vi "Execute PID Controllers.vi"(8 "error in (no error)":errorcluster, 11 "State Variables in":T1 {"Config"."Config"."Industrial Settings"."Write Refs"."Data Reference" format="%.0x"; "Config"."Config"."Industrial Settings"."Read Refs"."Data Reference" format="%.0x"; "Config"."Config"."PID Settings"."Read Refs"."Data Reference" format="%.0x"; "Config"."Config"."PID Settings"."Write Refs"."Data Reference" format="%.0x"}) -> (0 "error out":errorcluster, 3 "State Variables out":T1 {"Config"."Config"."Industrial Settings"."Write Refs"."Data Reference" format="%.0x"; "Config"."Config"."Industrial Settings"."Read Refs"."Data Reference" format="%.0x"; "Config"."Config"."PID Settings"."Read Refs"."Data Reference" format="%.0x"; "Config"."Config"."PID Settings"."Write Refs"."Data Reference" format="%.0x"})   [LabVIEW 2019, in "Control Addon Engine.lvlib"]
uses:
  Control Addon Engine.lvlib
  Types/RT Driver State Variables.ctl
  <vilib>/NI/NIVS Inline Async API/_VS Inline Async API/VS Inline Async API/VS Inline Async API.lvclass
  Types/RT Configuration.ctl
  Addon Shared/Types/Gain Schedule.ctl
  Addon Shared/Types/Compiled Settings.ctl
  Addon Shared/Types/Compiled PID Settings.ctl
  <vilib>/NI VeriStand/Custom Device API/Block Data Reference.ctl
  <vilib>/NI VeriStand/Custom Device API/Data Reference.ctl
  Addon Shared/Types/Compiled Industrial Settings.ctl
  Addon Shared/Types/Compiled Industrial Parameters.ctl
  <vilib>/addons/control/pid/pid.llb/PID Parameter Manager (DBL Array).vi
  <vilib>/addons/control/pid/pid.llb/PID Derivative Action Buffered (DBL Array).vi
  <vilib>/addons/control/pid/pid.llb/PID Get Advanced Error (DBL Array).vi
  <vilib>/addons/control/pid/pid.llb/PID Integral Action Buffered (DBL Array).vi
  <vilib>/addons/control/pid/pid.llb/PID Resize 1D Array.vi
  <vilib>/addons/control/pid/pid.llb/PID Get Advanced Error (DBL).vi
  <vilib>/NI VeriStand/Custom Device API/Global Data Refs.vi
  <vilib>/addons/control/pid/pid.llb/PID Gain Schedule.vi
  <vilib>/addons/control/pid/pid.llb/PID Gain Schedule (DBL).vi
  <vilib>/addons/control/pid/pid.llb/PID Output Rate Limiter (DBL Array).vi
  <vilib>/NI VeriStand/Custom Device API/Custom Device API.lvlib
  <vilib>/addons/control/pid/NI_PID_pid.lvlib
  Addon Shared/Control Addon Shared.lvlib
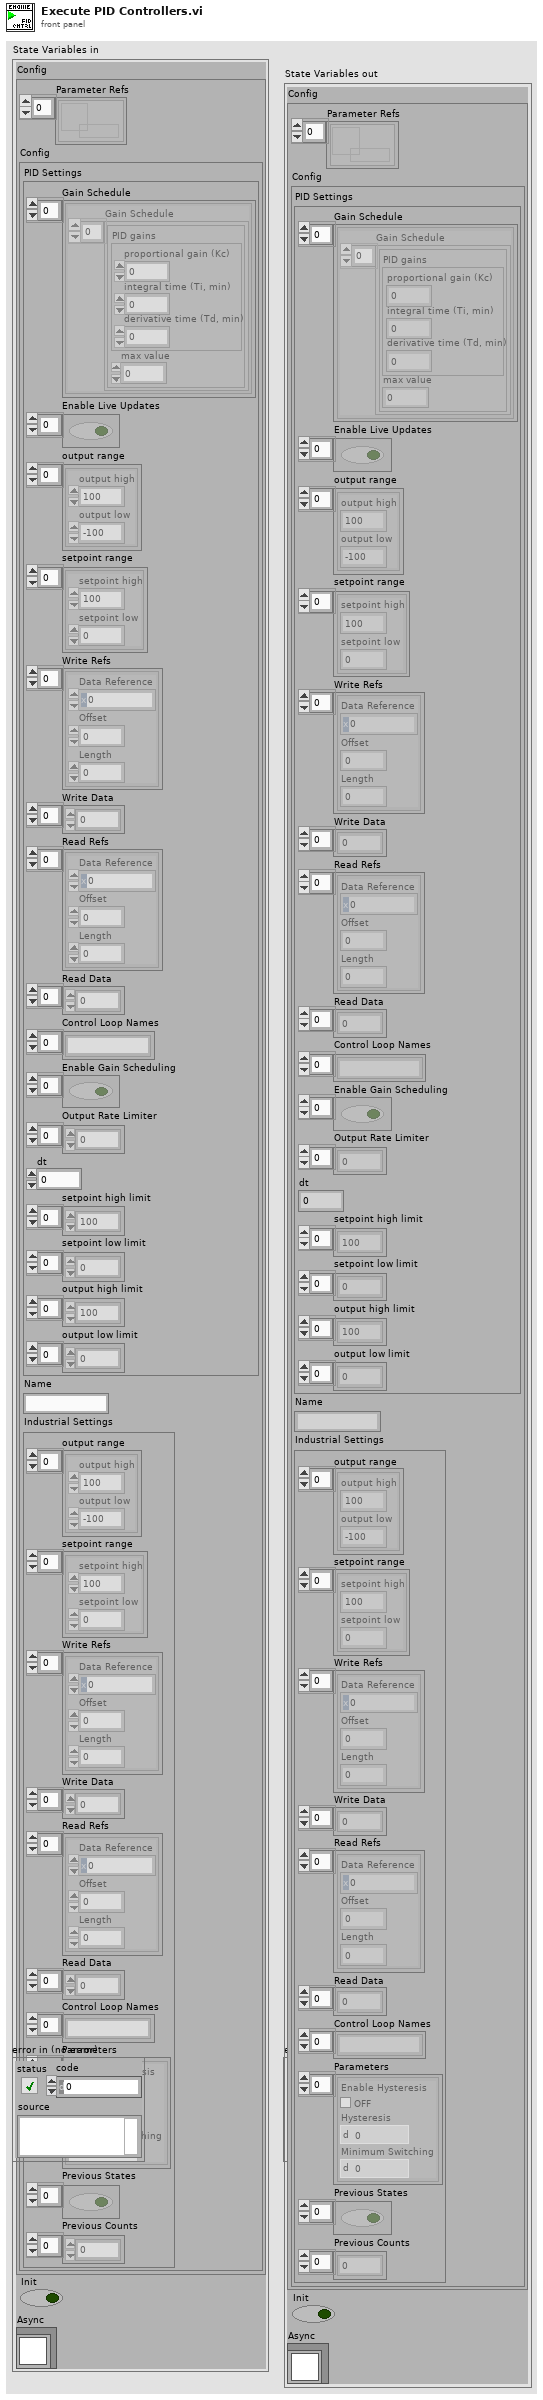
[diagram p1: front panel]
types:
  T1 = typedef "Control Addon Engine.lvlib/RT Driver State Variables.ctl" = cluster{"Config":T2, "Init":bool, "Async":refnum<class "VS Inline Async API.lvclass">}
  T2 = typedef "Control Addon Engine.lvlib/RT Configuration.ctl" = cluster{"Parameter Refs":refnum<data-value>[], "Config":T3}
  T3 = typedef "Control Addon Shared.lvlib/Compiled Settings.ctl" = cluster{"PID Settings":T4, "Name":string, "Industrial Settings":T8}
  T4 = typedef "Control Addon Shared.lvlib/Compiled PID Settings.ctl" = cluster{"Gain Schedule":T5[], "Enable Live Updates":bool[], "output range":cluster{"output high":dbl, "output low":dbl}[], "setpoint range":cluster{"setpoint high":dbl, "setpoint low":dbl}[], "Write Refs":T6[], "Write Data":dbl[], "Read Refs":T6[], "Read Data":dbl[], "Control Loop Names":string[], "Enable Gain Scheduling":bool[], "Output Rate Limiter":dbl[], "dt":dbl, "setpoint high limit":dbl[], "setpoint low limit":dbl[], "output high limit":dbl[], "output low limit":dbl[]}
  T5 = typedef "Control Addon Shared.lvlib/Gain Schedule.ctl" = cluster{"Gain Schedule":cluster{"PID gains":cluster{"proportional gain (Kc)":dbl, "integral time (Ti, min)":dbl, "derivative time (Td, min)":dbl}, "max value":dbl}[]}
  T6 = typedef "Custom Device API.lvlib/Block Data Reference.ctl" = cluster{"Data Reference":T7, "Offset":u64, "Length":u64}
  T7 = typedef "Custom Device API.lvlib/Data Reference.ctl" = i32
  T8 = typedef "Control Addon Shared.lvlib/Compiled Industrial Settings.ctl" = cluster{"output range":cluster{"output high":dbl, "output low":dbl}[], "setpoint range":cluster{"setpoint high":dbl, "setpoint low":dbl}[], "Write Refs":T6[], "Write Data":dbl[], "Read Refs":T6[], "Read Data":dbl[], "Control Loop Names":string[], "Parameters":T9[], "Previous States":bool[], "Previous Counts":u64[]}
  T9 = typedef "Control Addon Shared.lvlib/Compiled Industrial Parameters.ctl" = cluster{"Enable Hysteresis":bool, "Hysteresis":dbl, "Minimum Switching":u64}
  T10 = cluster{"setpoint high":dbl, "setpoint low":dbl}[]
  T11 = cluster{"proportional gain (Kc)":dbl, "integral time (Ti, min)":dbl, "derivative time (Td, min)":dbl}[]
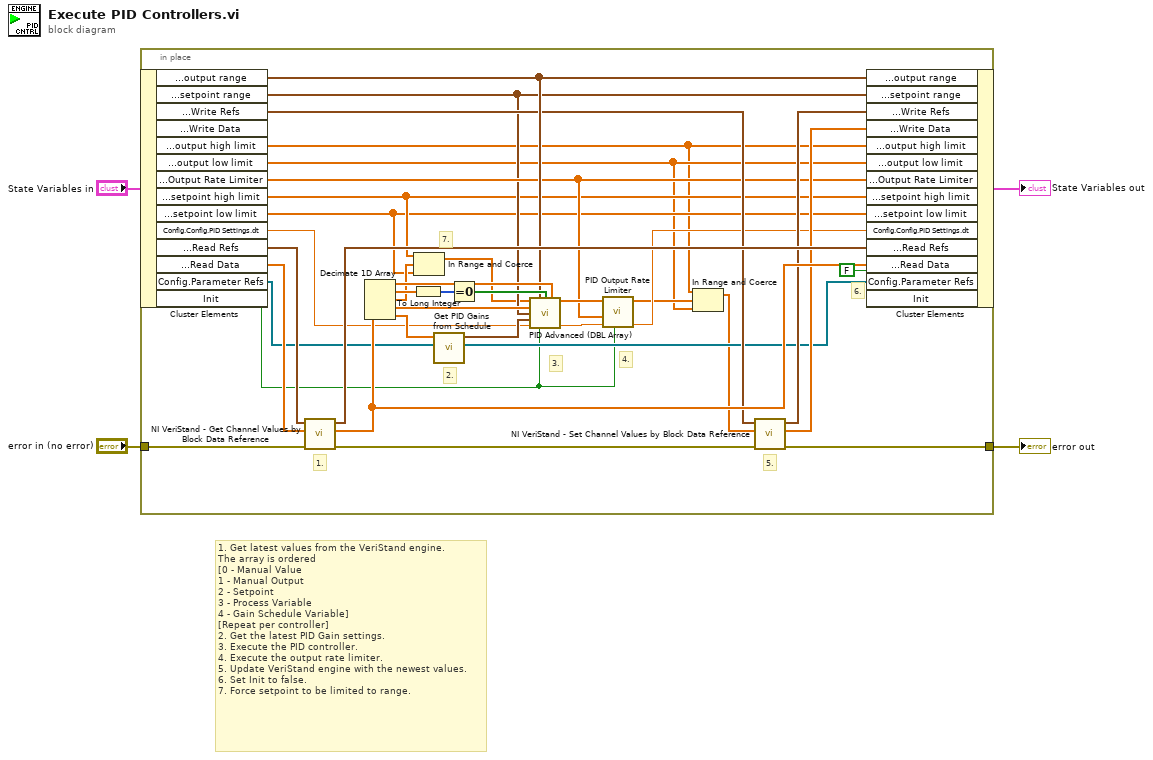
[diagram p0: block diagram]
diagram:
  # "1. Get latest values from the VeriStand engine.\nThe array is ordered\n[0 - Manual Value\n1 - Manual Output\n2 - Setpoint\n3 - Process Variable\n4 - Gain Schedule Variable]\n[Repeat per controller]\n2. Get the latest PID Gain settings.\n3. Execute the PID controller.\n4. Execute the output rate limiter.\n5. Update VeriStand engine with the newest values.\n6. Set Init to false.\n7. Force setpoint to be limited to range."
  n1 = in-place {
    in-place-border: "error in (no error)" -> [w40]
    in-place-border: [w27] -> w4
    # "7."
    # "6."
    # "5."
    # "4."
    # "3."
    # "2."
    # "1."
    n2 = in-place-cluster #1("State Variables in") -> ("Config.Config.PID Settings.output range"=w28:cluster{"output high":dbl, "output low":dbl}[], "Config.Config.PID Settings.setpoint range"=w13:T10, "Config.Config.PID Settings.Write Refs"=w26:T6[], "Config.Config.PID Settings.output high limit"=w5:dbl[], "Config.Config.PID Settings.output low limit"=w6:dbl[], "Config.Config.PID Settings.Output Rate Limiter"=w19:dbl[], "Config.Config.PID Settings.setpoint high limit"=w10:dbl[], "Config.Config.PID Settings.setpoint low limit"=w9:dbl[], "Config.Config.PID Settings.dt"=w17:dbl, "Config.Config.PID Settings.Read Refs"=w39:T6[], "Config.Config.PID Settings.Read Data"=w38:dbl[], "Config.Parameter Refs"=w22:refnum<data-value>[], "Init"=w15:bool)  [unwired: 1 out]
    n3 = call <vilib>:"NI VeriStand - Get Channel Values by Block Data Reference.vi"("error in (no error)"=w40, "Values Array in"=w38, "Block Data Ref"=w39) -> ("error out"=w35:errorcluster, "Values Array out"=w34:dbl[], "Block Data Ref dup"=w36:T6[])  [unwired: 6 in]
    n4 = Decimate 1D Array(w34) -> (w33:dbl[], w31:dbl[], w12:dbl[], w30:dbl[], w23:dbl[])
    n5 = To Long Integer(number=w31) -> (32bit integer=w37:i32[])
    n6 = In Range and Coerce(upper limit=w10, x=w12, lower limit=w9) -> (coerced(x)=w11:dbl[])  [unwired: 1 out]
    n7 = call "Get PID Gains from Schedule.vi"("Parameter Refs"=w22, "Gain Schedule Value"=w23) -> ("Parameter Refs"=w21:refnum<data-value>[], "PID"=w29:T11)  [unwired: 8 in]
    n8 = Equal To 0?(x=w37) -> (x = 0?=w32:bool[])
    n9 = call <vilib>:"PID Advanced (DBL Array).vi"("setpoint"=w11, "output range"=w28, "auto? (T)"=w32, "manual control"=w33, "process variable"=w30, "setpoint range"=w13, "PID gains"=w29, "dt (s)"=w17, "reinitialize? (F)"=w15) -> ("output"=w20:dbl[], "dt out (s)"=w18:dbl)  [unwired: 5 in]
    n10 = call-poly <vilib>:"PID Output Rate Limiter.vi"("reinitialize? (F)"=w15, "dt (s)"=w18, "output rate (EGU/min)"=w19, "input (controller output)"=w20) -> ("dt out (s)"=w16:dbl, "output"=w8:dbl[])  [unwired: 4 in]
    n11 = In Range and Coerce(upper limit=w5, x=w8, lower limit=w6) -> (coerced(x)=w7:dbl[])  [unwired: 1 out]
    n12 = call <vilib>:"NI VeriStand - Set Channel Values by Block Data Reference.vi"("error in (no error)"=w35, "Values Array in"=w7, "Block Data Ref"=w26) -> ("error out"=w27:errorcluster, "Values Array out"=w25:dbl[], "Block Data Ref dup"=w24:T6[])  [unwired: 6 in]
    n13 = in-place-cluster #1("Config.Config.PID Settings.output range"=w28, "Config.Config.PID Settings.setpoint range"=w13, "Config.Config.PID Settings.Write Refs"=w24, "Config.Config.PID Settings.Write Data"=w25, "Config.Config.PID Settings.output high limit"=w5, "Config.Config.PID Settings.output low limit"=w6, "Config.Config.PID Settings.Output Rate Limiter"=w19, "Config.Config.PID Settings.setpoint high limit"=w10, "Config.Config.PID Settings.setpoint low limit"=w9, "Config.Config.PID Settings.dt"=w16, "Config.Config.PID Settings.Read Refs"=w36, "Config.Config.PID Settings.Read Data"=w34, "Config.Parameter Refs"=w21, "Init"=FALSE) -> (→"State Variables out":T1)
  }
  "error out" <- w4
